vi "Sequence-StepComplete.vi"(0 "MCListbox Refnum":refnum<vi>, 5 "Step Feedback":T1, 11 "error in (no error)":errorcluster, 12 "length (rest)":i32) -> (4 "MCListbox Refnum(dup)":refnum<vi>, 15 "error out":errorcluster)   [LabVIEW 2020, in "CSMStand(Lite).lvlib"]
uses:
  CSMStand(Lite).lvlib
  <vilib>/Utility/miscctls.llb/LVRowAndColumnTypeDef.ctl
  d146a9cb-ae7a-4dd4-bb46-4eefd7c37fd3.vi
  <userlib>/_NEVSTOP/Communicable State Machine(CSM)/addons/API-String-Arugments-Support/_Support/Data To API String Arguments.vi
  <userlib>/NEVSTOP-Programming-Palette/Dialog & Interface/_support/Autosize All MultiListbox Columns (Uniform Text)_nevstop.vi
panel:
  # "Connector Pane"
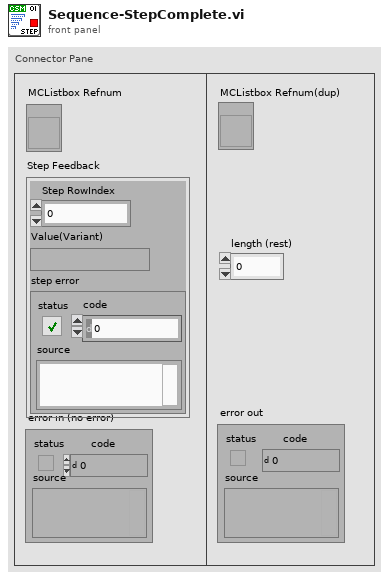
[diagram p1: front panel]
types:
  T1 = cluster{"Step RowIndex":i32, "Value(Variant)":variant, "step error":errorcluster}
  T2 = typedef "LVRowAndColumnTypeDef.ctl" = cluster{"Row":i32, "Column":i32}
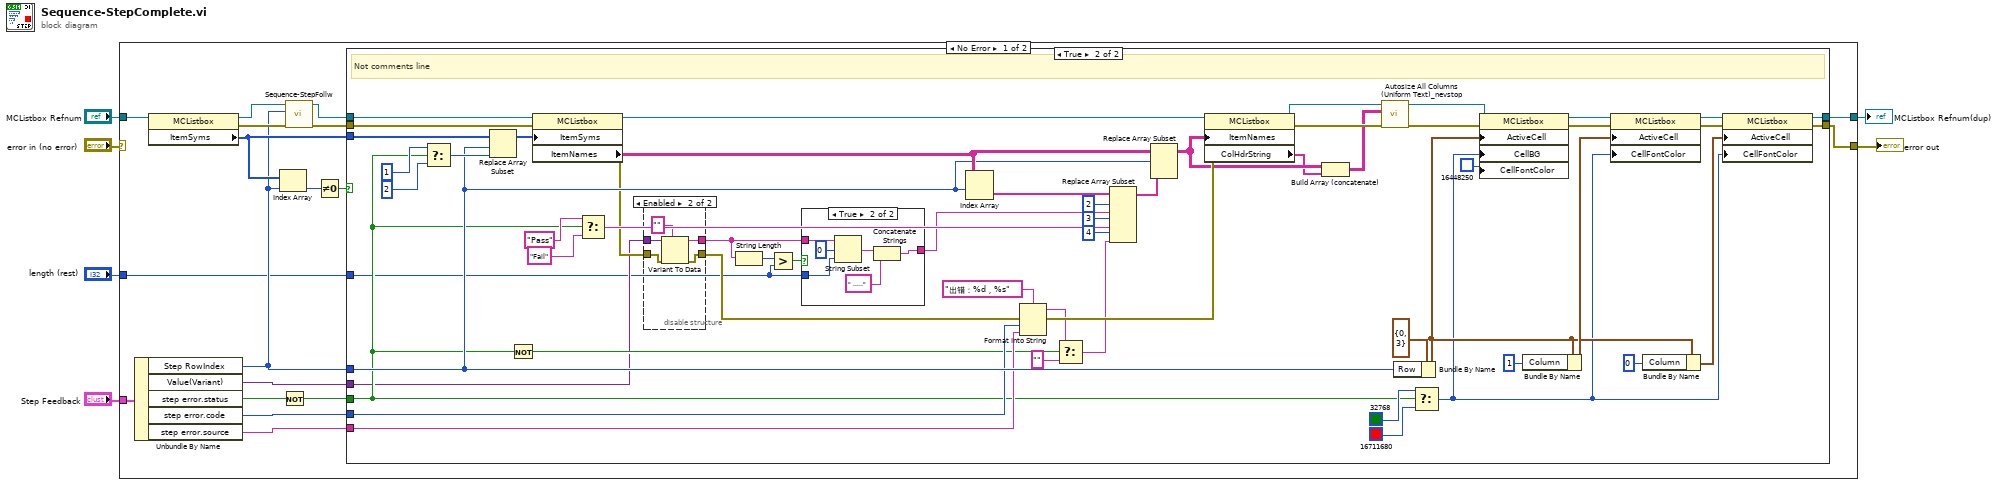
[diagram p0: block diagram]
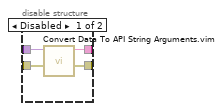
[diagram p3: hidden frame]
diagram:
  n1 = case shown="No Error" "error in (no error)" {
    selector: "error in (no error)" -> [_ w102]
    tunnel: [w22 w102] -> w6
    tunnel: "MCListbox Refnum" -> [w24 w101]
    tunnel: [w23 w101] -> w3
    tunnel: "Step Feedback" -> [w16 _]
    tunnel: "length (rest)" -> [w7 _]
    frame No Error {
      n2 = Unbundle By Name(w16) -> ("Step RowIndex"=w8:i32, "Value(Variant)"=w18:variant, "step error.status"=w17:bool, "step error.code"=w15:i32, "step error.source"=w14:string)
      n3 = property class="MCListbox"(reference=w24) -> (reference out=w10:refnum<vi>, error out=w12:errorcluster, "ItemSyms"=w21:i32[])  [unwired: 1 in]
      n4 = Index Array(array=w21, index=w8) -> (element=w20:i32)
      n5 = Not(x=w17) -> (.not. x?=w13:bool)
      n6 = call "Sequence-StepFollw.vi"("error in (no error)"=w12, "Row Index"=w8, "MCListbox Refnum"=w10) -> ("error out"=w11:errorcluster, "MCListbox Refnum(dup)"=w9:refnum<vi>)  [unwired: 7 in]
      n7 = Not Equal To 0?(x=w20) -> (x != 0?=w19:bool)
      n8 = case shown="True" w19 {
        tunnel: [w26 w40] -> w23
        tunnel: [w25 w37] -> w22
        tunnel: w9 -> [w26 w83]
        tunnel: w11 -> [w25 w78]
        tunnel: w13 -> [_ w52]
        tunnel: w21 -> [_ w74]
        tunnel: w8 -> [_ w66]
        tunnel: w18 -> [_ w32]
        tunnel: w15 -> [_ w55]
        tunnel: w14 -> [_ w54]
        tunnel: w7 -> [_ w28]
        frame False {
        }
        frame True {
          # "Not comments line"
          n9 = Select(t=1 ("Step RowIndex"), s=w52, f=2 ("Step RowIndex")) -> (s? t:f=w80:i32)
          n10 = Replace Array Subset(array=w74, new element=w80, index=w66) -> (w77:i32[])
          n11 = Not(x=w52) -> (.not. x?=w48:bool)
          n12 = property class="MCListbox"(reference=w83, error in=w78, "ItemSyms"=w77) -> (reference out=w79:refnum<vi>, error out=w63:errorcluster, "ItemNames"=w67:string[][])
          n13 = Select(t="Pass", s=w52, f="Fail") -> (s? t:f=w70:string)
          n14 = disable-structure shown="Enabled" {
            disable-tunnel: w63 -> [w88 w91]
            disable-tunnel: [w87 w90] -> w57
            disable-tunnel: w32 -> [w86 w92]
            disable-tunnel: [w85 w93] -> w30
            frame Disabled {
              n15 = call "Convert Data To API String Arguments.vim"("error in (no error)"=w88, "Data"=w86) -> ("error out"=w87:errorcluster, "API String"=w85:string)  [unwired: 6 in]
            }
            frame Enabled {
              n16 = Variant To Data(error in=w91, type="", Variant=w92) -> (data=w93:string, error out=w90:errorcluster)
            }
          }
          n17 = String Length(string=w30) -> (length=w29:i32)
          n18 = Greater?(x=w29, y=w28) -> (0:w27:bool)
          n19 = case shown="True" w27 {
            tunnel: [w94 w96] -> w31
            tunnel: w30 -> [w94 w98]
            tunnel: w28 -> [_ w97]
            frame False {
            }
            frame True {
              n20 = String Subset(string=w98, offset (0)=0, length (rest)=w97) -> (substring=w99:string)
              n21 = Concatenate Strings(w99, " ....." ("string")) -> (w96:string)
            }
          }
          n22 = Index Array(array=w67, index (row)=w66) -> (element=w73:string[])  [unwired: 1 in]
          n23 = Format Into String(format string="出错：%d，%s", error in=w57, w55, w54) -> (resulting string=w51:string, error out=w56:errorcluster)  [unwired: 1 in]
          n24 = Select(t=w51, s=w48, f="") -> (s? t:f=w49:string)
          n25 = Replace Array Subset(array=w73, new element #1=w31, index #1=2 ("index"), new element #2=w70, index #2=3 ("index"), new element #3=w49, index #3=4 ("index")) -> (w65:string[])
          n26 = Replace Array Subset(array=w67, new element=w65, index (row)=w66) -> (w47:string[][])  [unwired: 1 in]
          n27 = property class="MCListbox"(reference=w79, error in=w56, "ItemNames"=w47) -> (reference out=w60:refnum<vi>, error out=w62:errorcluster, "ColHdrString"=w46:string[])
          n28 = Build Array (concatenate)(w47, w46) -> (w45:string[][])
          n29 = call-poly <userlib>:"Autosize All Columns (Uniform Text)_nevstop.vi"("error in (no error)"=w62, "Array"=w45, "Control in"=w60) -> ("error out"=w61:errorcluster, "Control in"=w59:refnum<vi>)  [unwired: 7 in]
          n30 = Bundle By Name(cluster=T2 {"Row"=0, "Column"=3} ("Active Cell:Active Cell"), "Row"=w66) -> (w36:T2)
          n31 = Select(t=u32 32768 ("Active Cell:Cell Font:Color"), s=w52, f=u32 16711680 ("Active Cell:Cell Font:Color")) -> (s? t:f=w34:u32)
          n32 = property class="MCListbox"(reference=w59, error in=w61, "ActiveCell"=w36, "CellBG"=w34, "CellFontColor"=u32 16448250 ("Active Cell:Cell Font:Color")) -> (reference out=w44:refnum<vi>, error out=w43:errorcluster)
          n33 = Bundle By Name(cluster=w36, "Column"=1) -> (w41:T2)
          n34 = property class="MCListbox"(reference=w44, error in=w43, "ActiveCell"=w41, "CellFontColor"=w34) -> (reference out=w39:refnum<vi>, error out=w38:errorcluster)
          n35 = Bundle By Name(cluster=w36, "Column"=0) -> (w33:T2)
          n36 = property class="MCListbox"(reference=w39, error in=w38, "ActiveCell"=w33, "CellFontColor"=w34) -> (reference out=w40:refnum<vi>, error out=w37:errorcluster)
        }
      }
    }
    frame Error {
    }
  }
  "error out" <- w6
  "MCListbox Refnum(dup)" <- w3
